vi "PSVCH_Load Thread.vi"(5 "Close VIRef? (F)":bool, 6 "Type":u16(ring)=8 items=["Single"=0, "Reentrant"=8], 7 "Open FP? (F)":bool, 8 "Error In":errorcluster caption="错误输入（无错误）", 9 "Control Value":variant, 10 "Control Name":string="Parameter", 11 "VIRef":refnum<vi>) -> (0 "Error Out":errorcluster caption="错误输入（无错误）", 3 "VIRef":refnum<vi>)   [LabVIEW 2016]
panel:
  # "Data In"
  # "Data Out"
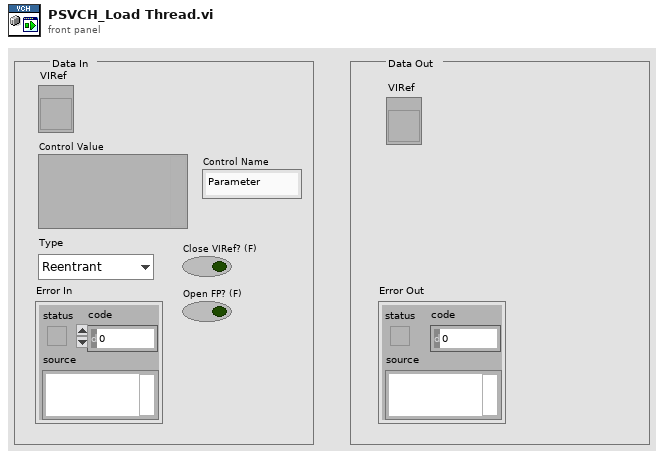
[diagram p1: front panel]
types:
  T1 = enum32{"Invalid", "Standard", "Closed", "Hidden", "Minimized", "Maximized"}
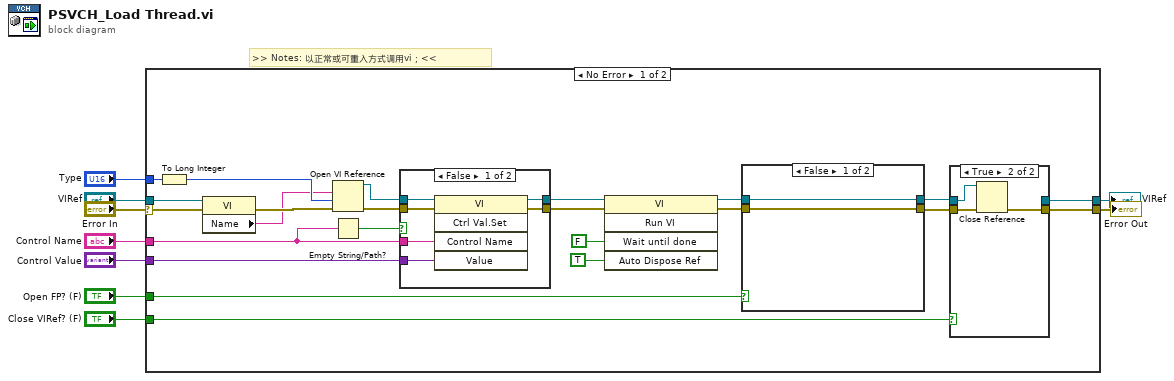
[diagram p0: block diagram]
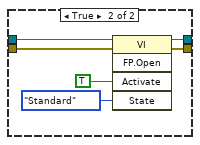
[diagram p3: hidden frame]
diagram:
  # ">> Notes: 以正常或可重入方式调用vi；<<"
  n1 = case shown="No Error" "Error In" {
    selector: "Error In" -> [w13 w54]
    tunnel: [w16 w54] -> w8
    tunnel: "Type" -> [w32 _]
    tunnel: "Control Name" -> [w27 _]
    tunnel: "Control Value" -> [w26 _]
    tunnel: "Open FP? (F)" -> [w19 _]
    tunnel: "Close VIRef? (F)" -> [w15 _]
    tunnel: [w14 _] -> w2
    tunnel: "VIRef" -> [w10 _]
    frame No Error {
      n2 = To Long Integer(number=w32) -> (32bit integer=w31:i32)
      n3 = property class="VI"(reference=w10, error in=w13) -> (error out=w12:errorcluster, "Name"=w11:string)  [unwired: 1 out]
      n4 = Open VI Reference(vi path=w11, options=w31, error in (no error)=w12) -> (vi reference=w28:refnum<vi>, error out=w30:errorcluster)  [unwired: 3 in]
      n5 = Empty String/Path?(string/path=w27) -> (empty?=w29:bool)
      n6 = case shown="False" w29 {
        tunnel: w28 -> [w51 w53]
        tunnel: [w50 w53] -> w23
        tunnel: [w49 w52] -> w22
        tunnel: w30 -> [w48 w52]
        tunnel: w27 -> [w47 _]
        tunnel: w26 -> [w46 _]
        frame False {
          n7 = invoke class="VI" method="Ctrl Val.Set"(reference=w51, error in=w48, "Control Name"=w47, "Value"=w46) -> (reference out=w50:refnum<vi>, error out=w49:errorcluster)  [unwired: 1 in, 3 out]
        }
        frame True {
        }
      }
      n8 = invoke class="VI" method="Run VI"(reference=w23, error in=w22, "Wait until done"=FALSE, "Auto Dispose Ref"=TRUE ("Auto Dispose Reference")) -> (reference out=w20:refnum<vi>, error out=w21:errorcluster)  [unwired: 1 in, 3 out]
      n9 = case shown="False" w19 {
        tunnel: w21 -> [w38 w41]
        tunnel: w20 -> [w39 w43]
        tunnel: [w39 w42] -> w17
        tunnel: [w38 w40] -> w18
        frame False {
        }
        frame True {
          n10 = invoke class="VI" method="FP.Open"(reference=w43, error in=w41, "Activate"=TRUE ("激活？"), "State"=T1."Standard" ("状态")) -> (reference out=w42:refnum<vi>, error out=w40:errorcluster)  [unwired: 1 in, 3 out]
        }
      }
      n11 = case shown="True" w15 {
        tunnel: w18 -> [w34 w37]
        tunnel: w17 -> [w33 w36]
        tunnel: [w34 w35] -> w16
        tunnel: [w33 _] -> w14
        frame False {
        }
        frame True {
          n12 = Close Reference(reference=w36, error in (no error)=w37) -> (error out=w35:errorcluster)
        }
      }
    }
    frame Error {
    }
  }
  "Error Out" <- w8
  "VIRef" <- w2
